vi "networkstreamRead.vi"() -> (2 "data out":cluster{dbl, dbl}[](array[cluster]))   [LabVIEW 2014]
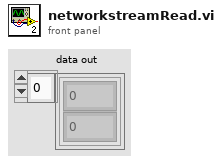
[diagram p1: front panel]
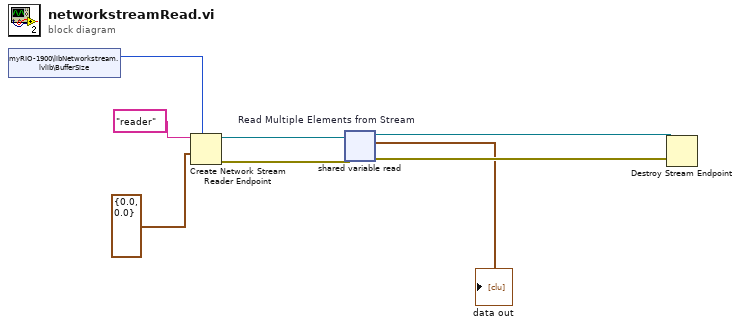
[diagram p0: block diagram]
diagram:
  n1 = shared-variable "myRIO-1900\\libNetworkstream.lvlib\\BufferSize"() -> (w1:i32)  [unwired: 1 in, 1 out]
  n2 = Create Network Stream Reader Endpoint(7:w1, 9:cluster{dbl, dbl} {0.0, 0.0}, 11:"reader" ("reader name")) -> (0:w7:errorcluster, 3:w8:refnum<k21>)  [unwired: 4 in]
  n3 = shared-variable-read "Read Multiple Elements from Stream"(w8, w7) -> (w3:refnum<k21>, w4:errorcluster, →"data out":cluster{dbl, dbl}[])  [unwired: 2 in, 1 out]
  n4 = Destroy Stream Endpoint(8:w4, 11:w3) -> ()  [unwired: 1 out]
